vi "getMeasurementTimingBudget.vi"(8 "error in":errorcluster, 10 "Slave Address (7-bit)":u8, 11 "I2C Ref In":T3) -> (0 "error out":errorcluster, 2 "budget_us":u32, 3 "I2C Ref Out":T3)   [LabVIEW 2018]
uses:
  <vilib>/myRIO/Instrument Drivers/Onboard IO/I2C/typedefs/I2C Reference.ctl
  <vilib>/myRIO/Common/Instrument Driver Framework/Utilities/typedefs/myRIO Generic Hardware Reference.ctl
  <vilib>/myRIO/Common/Instrument Driver Framework/Utilities/typedefs/Hardware Version Enum.ctl
  <vilib>/myRIO/Common/Instrument Driver Framework/Utilities/typedefs/myRIO v1.0 Reference.ctl
  <vilib>/myRIO/Common/Instrument Driver Framework/Utilities/typedefs/Generic FPGA Reference.ctl
  <vilib>/myRIO/Common/Instrument Driver Framework/myRIO v1.0/I2C/typedefs/I2C Channels Enum.ctl
  <vilib>/myRIO/Instrument Drivers/Onboard IO/I2C/typedefs/I2C Configuration.ctl
  <vilib>/myRIO/Instrument Drivers/Onboard IO/I2C/typedefs/I2C Transfer Rate.ctl
  <vilib>/myRIO/Instrument Drivers/Onboard IO/I2C/I2C.lvlib
panel:
  out "enables":T1
  out "timeouts":T2
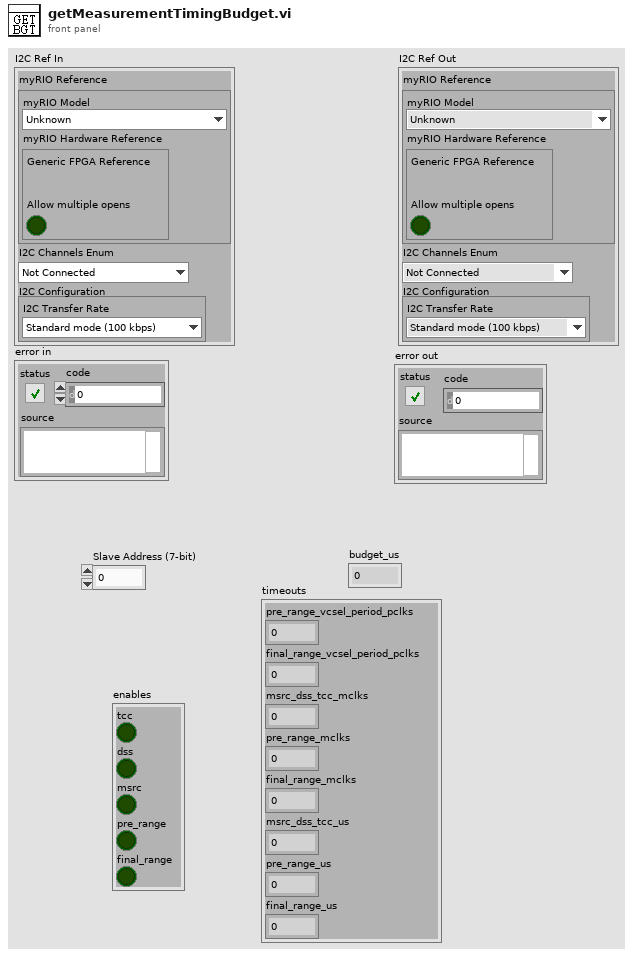
[diagram p1: front panel]
types:
  T1 = cluster{"tcc":bool, "dss":bool, "msrc":bool, "pre_range":bool, "final_range":bool}
  T2 = cluster{"pre_range_vcsel_period_pclks":u16, "final_range_vcsel_period_pclks":u16, "msrc_dss_tcc_mclks":u16, "pre_range_mclks":u16, "final_range_mclks":u16, "msrc_dss_tcc_us":u32, "pre_range_us":u32, "final_range_us":u32}
  T3 = typedef "I2C.lvlib/I2C Reference.ctl" = cluster{"myRIO Reference":T4, "I2C Channels Enum":T8, "I2C Configuration":T9}
  T4 = typedef "myRIO Generic Hardware Reference.ctl" = cluster{"myRIO Model":T5, "myRIO Hardware Reference":T6}
  T5 = typedef "Hardware Version Enum.ctl" = enum16{"Unknown", "myRIO-1900", "myRIO-1950", "roboRIO", "NI ELVIS RIO CM", "ELVIS III"}
  T6 = typedef "myRIO v1.0 Reference.ctl" = cluster{"Generic FPGA Reference":T7, "Allow multiple opens":bool}
  T7 = typedef "Generic FPGA Reference.ctl" = refnum<k20>
  T8 = typedef "I2C Channels Enum.ctl" = enum16{"Not Connected", "A/I2C", "B/I2C", "I2C/I2C"}
  T9 = typedef "I2C.lvlib/I2C Configuration.ctl" = cluster{"I2C Transfer Rate":T10}
  T10 = typedef "I2C.lvlib/I2C Transfer Rate.ctl" = enum16{"Standard mode (100 kbps)", "Fast mode (400 kbps)"}
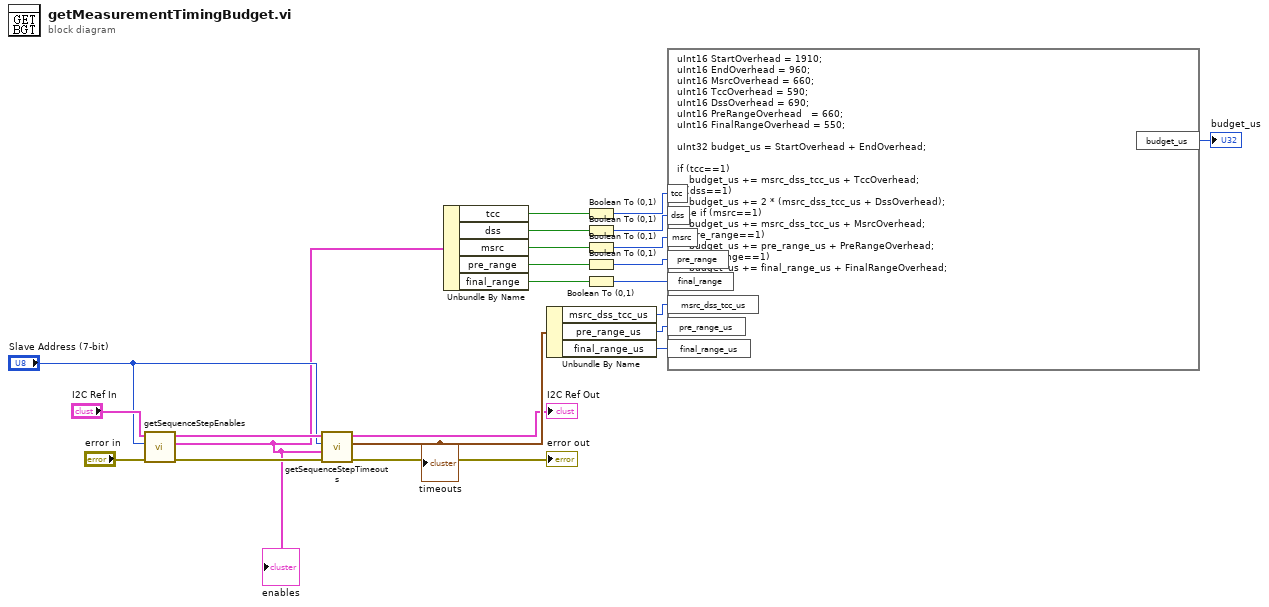
[diagram p0: block diagram]
diagram:
  n1 = call "getSequenceStepEnables.vi"("error in"="error in", "Slave Address (7-bit)"="Slave Address (7-bit)", "I2C Ref In"="I2C Ref In") -> ("error out"=w20:errorcluster, "enables"=w1:T1, "I2C Ref Out"=w21:T3)  [unwired: 6 in]
  "enables" <- w1
  n2 = call "getSequenceStepTimeouts.vi"("error in"=w20, "enables"=w1, "Slave Address (7-bit)"="Slave Address (7-bit)", "I2C Ref In"=w21) -> ("error out"=→"error out":errorcluster, "timeouts"=w8:T2, "I2C Ref Out"=→"I2C Ref Out":T3)  [unwired: 4 in]
  "timeouts" <- w8
  n3 = Unbundle By Name(w1) -> ("tcc"=w18:bool, "dss"=w17:bool, "msrc"=w16:bool, "pre_range"=w15:bool, "final_range"=w14:bool)
  n4 = Unbundle By Name(w8) -> ("msrc_dss_tcc_us"=w4:u32, "pre_range_us"=w3:u32, "final_range_us"=w2:u32)
  n5 = Boolean To (0,1)(Boolean=w18) -> (0, 1=w9:i16)
  n6 = Boolean To (0,1)(Boolean=w17) -> (0, 1=w10:i16)
  n7 = Boolean To (0,1)(Boolean=w16) -> (0, 1=w11:i16)
  n8 = Boolean To (0,1)(Boolean=w15) -> (0, 1=w12:i16)
  n9 = Boolean To (0,1)(Boolean=w14) -> (0, 1=w13:i16)
  n10 = formula code="uInt16 StartOverhead = 1910; \nuInt16 EndOverhead = 960;\nuInt16 MsrcOverhead = 660;\nuInt16 TccOverhead = 590;\nuInt16 DssOverhead = 690;\nuInt16 PreRangeOverhead   = 660;\nuInt16 FinalRangeOverhead = 550;\n\nuInt32 budget_us = StartOverhead + EndOverhead;\n\nif (tcc==1)\n    budget_us += msrc_dss_tcc_us + TccOverhead;\nif (dss==1)\n    budget_us += 2 * (msrc_dss_tcc_us + DssOverhead);\nelse if (msrc==1)\n    budget_us += msrc_dss_tcc_us + MsrcOverhead;\nif (pre_range==1)\n    budget_us += pre_range_us + PreRangeOverhead;\nif (final_range==1)\n    budget_us += final_range_us + FinalRangeOverhead;"("tcc"=w9, "dss"=w10, "msrc"=w11, "pre_range"=w12, "final_range"=w13, "msrc_dss_tcc_us"=w4, "pre_range_us"=w3, "final_range_us"=w2) -> ("budget_us"=→"budget_us":u32)
